vi "High Resolution Wait.vi"(8 "error in (no error)":errorcluster, 11 "wait time (s)":dbl) -> (0 "error out":errorcluster)   [LabVIEW 2017]
doc: "Waits the specified time. Use this VI when you need higher resolution of wait time than you can obtain with the Wait (ms) function. \n\nThe time resolution of this VI may vary with different operating systems and CPU types.\n\nUnlike the Wait (ms) function, this VI does not yield. If <b>wait time</b> is less than 1 to 2 ms, this VI polls in a tight loop. If <b>wait time</b> is greater than 1 to 2 ms, this VI polls in a tight loop for the last 1 to 2 ms."
uses:
  kernel32.dll
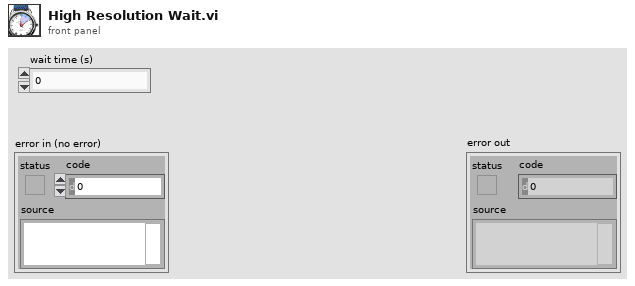
[diagram p1: front panel]
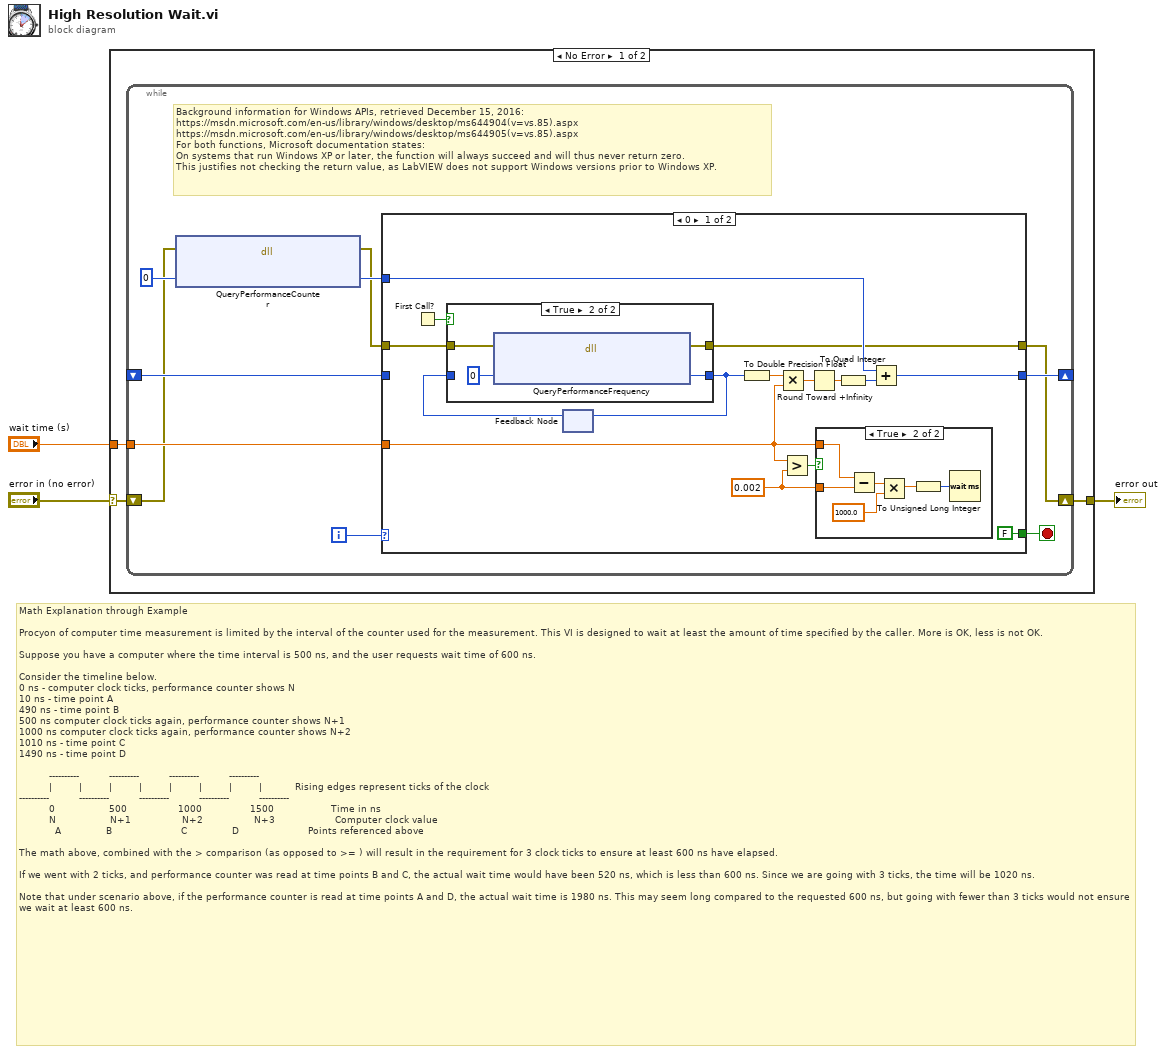
[diagram p0: block diagram]
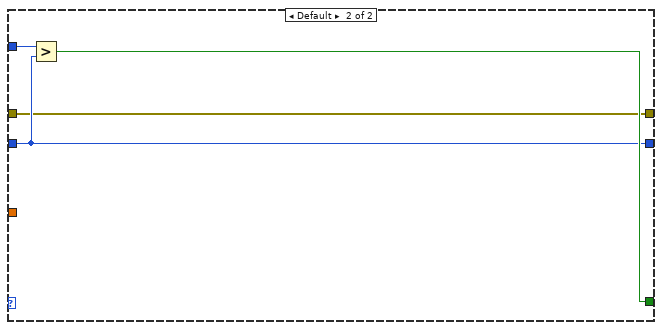
[diagram p4: hidden frame]
diagram:
  # "Math Explanation through Example\n\nProcyon of computer time measurement is limited by the interval of the counter used for the measurement. This VI is designed to wait at least the amount of time specified by the caller. More is OK, less is not OK.\n\nSuppose you have a computer where the time interval is 500 ns, and the user requests wait time of 600 ns.\n\nConsider the timeline below.\n0 ns - computer clock ticks, performance counter shows N\n10 ns - time point A\n490 ns - time point B\n500 ns computer clock ticks again, performance counter shows N+1\n1000 ns computer clock ticks again, performance counter shows N+2\n1010 ns - time point C\n1490 ns - time point D\n\n          ----------          ----------          ----------          ----------          \n          |         |         |         |         |         |         |         |           Rising edges represent ticks of the clock\n----------          ----------          ----------          ----------          ----------          \n          0                  500                 1000                1500                   Time in ns\n          N                  N+1                 N+2                 N+3                    Computer clock value\n            A               B                       C               D                       Points referenced above \n\nThe math above, combined with the > comparison (as opposed to >= ) will result in the requirement for 3 clock ticks to ensure at least 600 ns have elapsed.\n\nIf we went with 2 ticks, and performance counter was read at time points B and C, the actual wait time would have been 520 ns, which is less than 600 ns. Since we are going with 3 ticks, the time will be 1020 ns.\n\nNote that under scenario above, if the performance counter is read at time points A and D, the actual wait time is 1980 ns. This may seem long compared to the requested 600 ns, but going with fewer than 3 ticks would not ensure we wait at least 600 ns."
  n1 = case shown="No Error" "error in (no error)" {
    selector: "error in (no error)" -> [w5 w48]
    tunnel: "wait time (s)" -> [w6 _]
    tunnel: [w4 w48] -> w1
    frame No Error {
      n2 = while {
        shift-right: [w15] -> _
        shift-left: _ -> [w16]
        tunnel: w6 -> [w12]
        shift-right: [w7] -> w4
        shift-left: w5 -> [w9]
        i -> [w13]
        stop <- w14 stop-if-true
        # "Background information for Windows APIs, retrieved December 15, 2016:\nhttps://msdn.microsoft.com/en-us/library/windows/desktop/ms644904(v=vs.85).aspx\nhttps://msdn.microsoft.com/en-us/library/windows/desktop/ms644905(v=vs.85).aspx\nFor both functions, Microsoft documentation states:\nOn systems that run Windows XP or later, the function will always succeed and will thus never return zero.\nThis justifies not checking the return value, as LabVIEW does not support Windows versions prior to Windows XP."
        n3 = dll-call lib="kernel32.dll" fn="QueryPerformanceCounter"(error in=w9, "lpPerformanceCount"=i64 0) -> (error out=w8:errorcluster, "lpPerformanceCount"=w10:i64)  [unwired: 3 in, 1 out]
        n4 = case shown="0" w13 {
          tunnel: w16 -> [_ w46]
          tunnel: [w31 w46] -> w15
          tunnel: [FALSE w47] -> w14
          tunnel: w12 -> [w22 _]
          tunnel: w10 -> [w27 w45]
          tunnel: w8 -> [w18 w44]
          tunnel: [w17 w44] -> w7
          frame 0 {
            w28 = 0.002 ("y")
            n5 = First Call?() -> (First Call?: T/F=w21:bool)
            n6 = feedback #1() -> (w19:i64)  [unwired: 1 in]
            n7 = case shown="True" w21 {
              tunnel: w19 -> [w33 _]
              tunnel: [w33 w36] -> w20
              tunnel: w18 -> [w32 w35]
              tunnel: [w32 w34] -> w17
              frame False {
              }
              frame True {
                n8 = dll-call lib="kernel32.dll" fn="QueryPerformanceFrequency"(error in=w35, "lpFrequency"=i64 0) -> (error out=w34:errorcluster, "lpFrequency"=w36:i64)  [unwired: 3 in, 1 out]
              }
            }
            n9 = feedback-in #1(w20) -> ()
            n10 = To Double Precision Float(number=w20) -> (double precision float=w23:dbl)
            n11 = Multiply(x=w23, y=w22) -> (x*y=w26:dbl)
            n12 = Greater?(x=w22, y=w28) -> (0:w29:bool)
            n13 = Round Toward +Infinity(x=w26) -> (ceil(x): smallest int >= x=w25:dbl)
            n14 = case shown="True" w29 {
              tunnel: w22 -> [_ w39]
              tunnel: w28 -> [_ w38]
              frame False {
              }
              frame True {
                n15 = Subtract(x=w39, y=w38) -> (x-y=w43:dbl)
                n16 = Multiply(x=w43, y=1000.0) -> (x*y=w40:dbl)
                n17 = To Unsigned Long Integer(number=w40) -> (unsigned 32bit integer=w41:u32)
                n18 = Wait (ms)(milliseconds to wait=w41) -> ()  [unwired: 1 out]
              }
            }
            n19 = To Quad Integer(1:w25) -> (0:w24:i64)
            n20 = Add(x=w27, y=w24) -> (x+y=w31:i64)
          }
          frame Default {
            n21 = Greater?(x=w45, y=w46) -> (0:w47:bool)
          }
        }
      }
    }
    frame Error {
    }
  }
  "error out" <- w1
